vi "Sensors Modifications.vi"(1 "Sensors Global Values In":T1) -> (0 "Sensors Global Values Out":T1)   [LabVIEW 2013]
panel:
  in  "Sonar V/cm":dbl
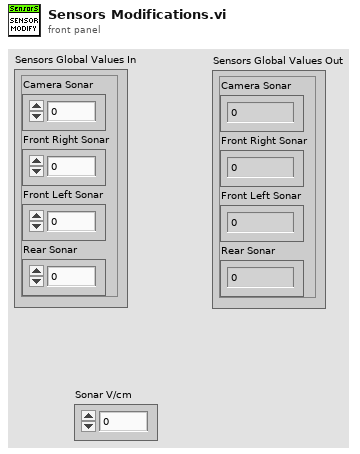
[diagram p1: front panel]
types:
  T1 = cluster{"Camera Sonar":dbl, "Front Right Sonar":dbl, "Front Left Sonar":dbl, "Rear Sonar":dbl}
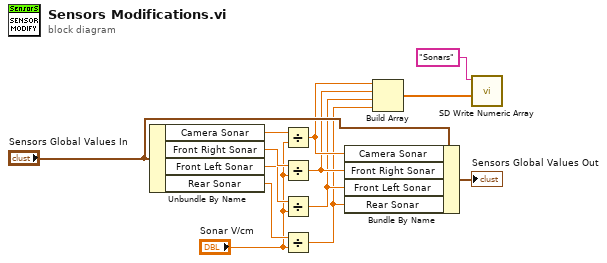
[diagram p0: block diagram]
diagram:
  n1 = Unbundle By Name("Sensors Global Values In") -> ("Camera Sonar"=w11:dbl, "Front Right Sonar"=w10:dbl, "Front Left Sonar"=w9:dbl, "Rear Sonar"=w8:dbl)
  n2 = Divide(x=w11, y="Sonar V/cm") -> (x/y=w4:dbl)
  n3 = Divide(x=w10, y="Sonar V/cm") -> (x/y=w3:dbl)
  n4 = Divide(x=w9, y="Sonar V/cm") -> (x/y=w2:dbl)
  n5 = Divide(x=w8, y="Sonar V/cm") -> (x/y=w1:dbl)
  n6 = Bundle By Name(cluster="Sensors Global Values In", "Camera Sonar"=w4, "Front Right Sonar"=w3, "Front Left Sonar"=w2, "Rear Sonar"=w1) -> (→"Sensors Global Values Out":T1)
  n7 = Build Array(w4, w3, w2, w1) -> (w5:dbl[])
  n8 = call <vilib>:"SD Write Numeric Array.vi"("Numeric Array"=w5, "Name"="Sonars") -> ()  [unwired: 8 in, 2 out]
